vi "PropertyChangedEventCallbackForScrollBar.vi"(4 "?":refnum<vi>, 5 "Event Data":cluster{"sender":refnum<k24>, "e":refnum<k24>}, 6 "Control Ref":refnum<k24>, 7 "Event Common Data":T1) -> ()   [LabVIEW 2018]
uses:
  D:/SVN/PM/sdk/AppSamples/LabVIEWSamples/trunk/Release/2018/Dependencies/PVCamNET.dll
  Dependencies/PVCamNET.dll
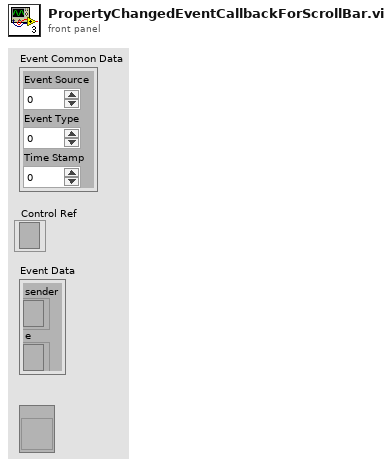
[diagram p1: front panel]
types:
  T1 = cluster{"Event Source":i32, "Event Type":u32, "Time Stamp":u32}
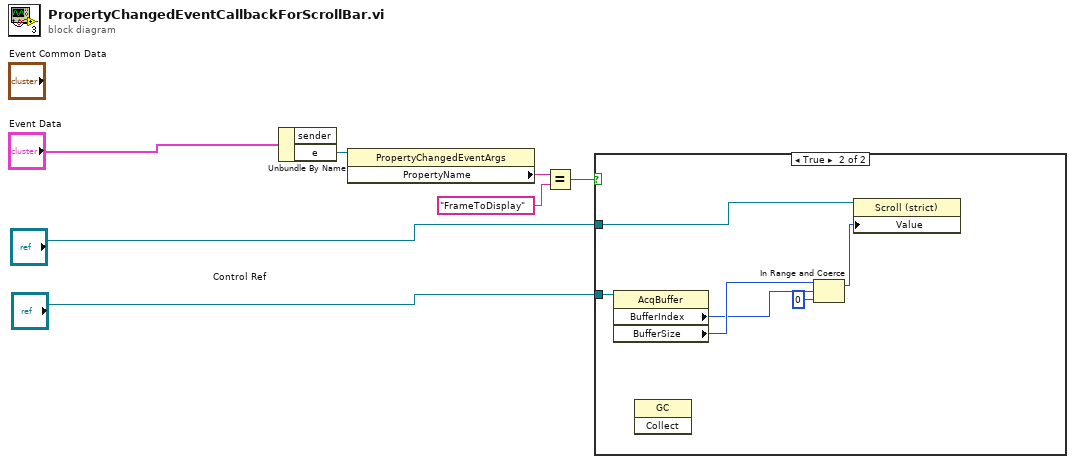
[diagram p0: block diagram]
diagram:
  n1 = Unbundle By Name("Event Data") -> ("e"=w7:refnum<k24>)  [unwired: 1 out]
  n2 = property class="PropertyChangedEventArgs"(reference=w7) -> ("PropertyName"=w6:string)  [unwired: 1 in, 2 out]
  n3 = Equal?(x=w6, y="FrameToDisplay") -> (x = y?=w4:bool)
  n4 = case shown="True" w4 {
    tunnel: "?" -> [_ w13]
    tunnel: "Control Ref" -> [_ w12]
    frame False {
    }
    frame True {
      n5 = property class="AcqBuffer"(reference=w12) -> ("BufferIndex"=w10:u32, "BufferSize"=w11:u32)  [unwired: 1 in, 2 out]
      n6 = invoke class="GC" method="Collect"() -> ()  [unwired: 3 in, 3 out]
      n7 = In Range and Coerce(upper limit=w11, x=w10, lower limit=0) -> (coerced(x)=w8:u32)  [unwired: 1 out]
      n8 = property class="Scroll (strict)"(reference=w13, "Value"=w8) -> ()  [unwired: 1 in, 2 out]
    }
  }
